vi "dtDeals.vi"(1 "n":u16=24, 5 "inDts":u8[](array[numeric]), 9 "rageMax":i32=24) -> (6 "values":dbl[](array[numeric]))   [LabVIEW 2015]
panel:
  out "数组":u16[](array[numeric])
  out "d":dbl
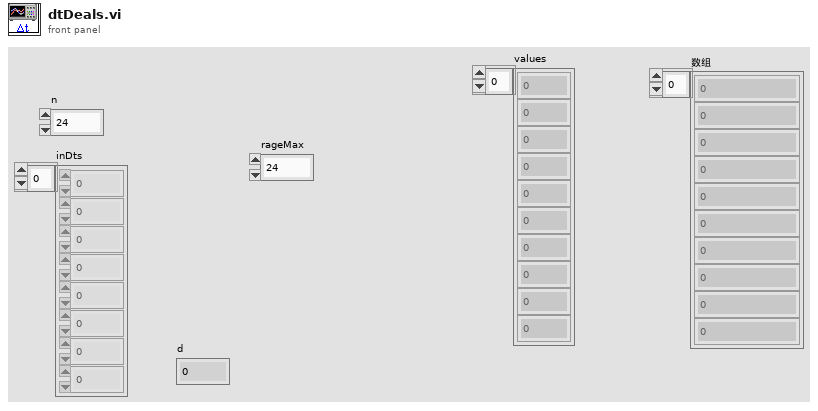
[diagram p1: front panel]
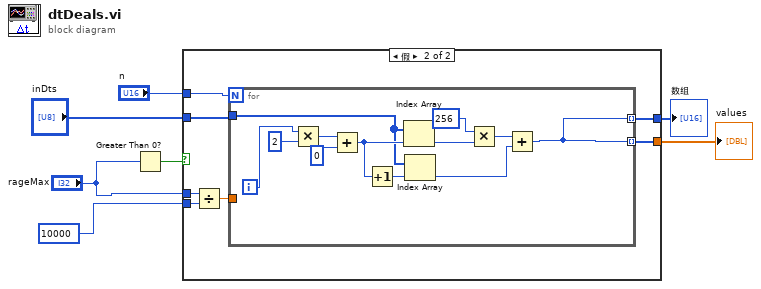
[diagram p0: block diagram]
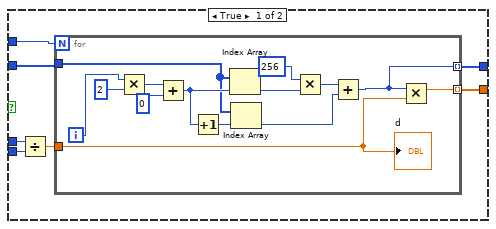
[diagram p2: hidden frame]
diagram:
  n1 = Greater Than 0?(x="rageMax") -> (x > 0?=w3:bool)
  n2 = case shown="假" w3 {
    tunnel: "n" -> [w14 w35]
    tunnel: "inDts" -> [w13 w34]
    tunnel: 10000 ("y") -> [w12 w33]
    tunnel: "rageMax" -> [w11 w32]
    tunnel: [w9 w30] -> w2
    tunnel: [w8 w29] -> w1
    frame True {
      n3 = Divide(x=w11, y=w12) -> (x/y=w10:dbl)
      n4 = for {
        N: w14 -> [_]
        tunnel: w13 -> [w18]
        tunnel: [w17] -> w9 mode=indexing
        tunnel: w10 -> [w16]
        tunnel: [w15] -> w8 mode=indexing
        i -> [w19]
        n5 = Multiply(x=w19, y=2) -> (x*y=w25:i32)
        n6 = Add(x=w25, y=0) -> (x+y=w27:i32)
        n7 = Increment(x=w27) -> (x+1=w28:i32)
        n8 = Index Array(array=w18, index=w27) -> (element=w20:u8)
        n9 = Index Array(array=w18, index=w28) -> (element=w23:u8)
        n10 = Multiply(x=u16 256, y=w20) -> (x*y=w22:u16)
        n11 = Add(x=w22, y=w23) -> (x+y=w15:u16)
        n12 = Multiply(x=w15, y=w16) -> (x*y=w17:dbl)
        "d" <- w16
      }
    }
    frame False {
      n13 = Divide(x=w32, y=w33) -> (x/y=w31:dbl)
      n14 = for {
        N: w35 -> [_]
        tunnel: w34 -> [w37]
        tunnel: [w36] -> w30 mode=indexing
        tunnel: w31 -> [_]
        tunnel: [w36] -> w29 mode=indexing
        i -> [w38]
        n15 = Multiply(x=w38, y=2) -> (x*y=w44:i32)
        n16 = Add(x=w44, y=0) -> (x+y=w46:i32)
        n17 = Increment(x=w46) -> (x+1=w47:i32)
        n18 = Index Array(array=w37, index=w46) -> (element=w39:u8)
        n19 = Index Array(array=w37, index=w47) -> (element=w42:u8)
        n20 = Multiply(x=u16 256, y=w39) -> (x*y=w41:u16)
        n21 = Add(x=w41, y=w42) -> (x+y=w36:u16)
      }
    }
  }
  "values" <- w2
  "数组" <- w1
